vi "Hardware - Trigger Timestamp.vi"(8 "error in (no error)":errorcluster) -> (0 "error out":errorcluster)   [LabVIEW 2010, in "Core SubVIs.lvlib"]
uses:
  Core SubVIs.lvlib
  <vilib>/DAQmx/write.llb/DAQmx Write (Digital Bool 1Line 1Point).vi
  <vilib>/daqmx/miscellaneous.llb/DAQmx Fill In Error Info.vi
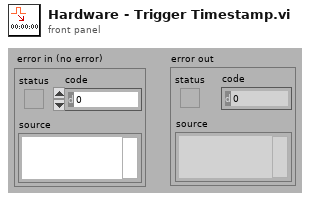
[diagram p1: front panel]
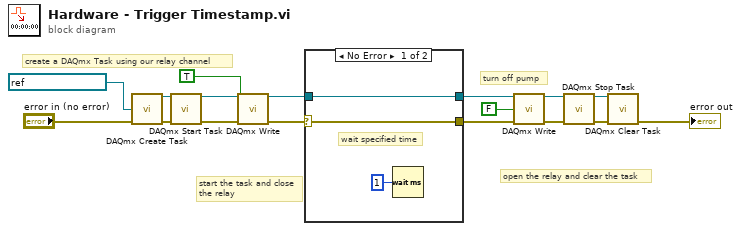
[diagram p0: block diagram]
diagram:
  # "open the relay and clear the task"
  # "start the task and close\nthe relay"
  # "create a DAQmx Task using our relay channel"
  # "turn off pump"
  n1 = call <vilib>:"DAQmx Create Task.vi"("global virtual channels"=refnum<k21> "EVENT_1_OUT", "error in"="error in (no error)") -> ("task out"=w16:refnum<k21>, "error out"=w15:errorcluster)  [unwired: 3 in, 9 out]
  n2 = call <vilib>:"DAQmx Start Task.vi"("task/channels in"=w16, "error in"=w15) -> ("task out"=w13:refnum<k21>, "error out"=w14:errorcluster)  [unwired: 12 out]
  n3 = call-poly <vilib>:"DAQmx Write.vi"("task/channels in"=w13, "data"=TRUE, "error in"=w14) -> ("task out"=w7:refnum<k21>, "error out"=w6:errorcluster)  [unwired: 1 in, 10 out]
  n4 = case shown="No Error" w6 {
    selector: w6 -> [w20 w21]
    tunnel: w7 -> [w19 w22]
    tunnel: [w20 w21] -> w5
    tunnel: [w19 w22] -> w4
    frame No Error {
      # "wait specified time"
      n5 = Wait (ms)(milliseconds to wait=u32 1) -> ()  [unwired: 1 out]
    }
    frame Error {
    }
  }
  n6 = call-poly <vilib>:"DAQmx Write.vi"("task/channels in"=w4, "data"=FALSE, "error in"=w5) -> ("task out"=w11:refnum<k21>, "error out"=w10:errorcluster)  [unwired: 1 in, 10 out]
  n7 = call <vilib>:"DAQmx Stop Task.vi"("task/channels in"=w11, "error in"=w10) -> ("task out"=w9:refnum<k21>, "error out"=w8:errorcluster)  [unwired: 12 out]
  n8 = call <vilib>:"DAQmx Clear Task.vi"("task in"=w9, "error in"=w8) -> ("error out"=→"error out":errorcluster)  [unwired: 13 out]
